vi "Status.vi"(2 "Big":bool, 3 "Little":bool) -> (0 "Cluster":T1)   [LabVIEW 2014]
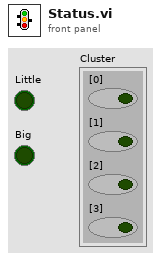
[diagram p1: front panel]
types:
  T1 = cluster{"[0]":bool, "[1]":bool, "[2]":bool, "[3]":bool}
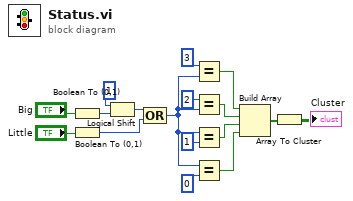
[diagram p0: block diagram]
diagram:
  n1 = Boolean To (0,1)(Boolean="Big") -> (0, 1=w4:i16)
  n2 = Boolean To (0,1)(Boolean="Little") -> (0, 1=w3:i16)
  n3 = Logical Shift(y=i16 1, x=w4) -> (x << y=w6:i16)
  n4 = Compound Arithmetic op=OR(w6, w3) -> (w16:i16)
  n5 = Equal?(x=i16 3, y=w16) -> (x = y?=w7:bool)
  n6 = Equal?(x=i16 2, y=w16) -> (x = y?=w8:bool)
  n7 = Equal?(x=w16, y=i16 1) -> (x = y?=w9:bool)
  n8 = Equal?(x=w16, y=i16 0) -> (x = y?=w10:bool)
  n9 = Build Array(w7, w8, w9, w10) -> (w12:bool[])
  n10 = Array To Cluster(array=w12) -> (cluster=→"Cluster":T1)
